vi "Clear All.vi"(8 "error in (no error)":errorcluster, 11 ".NET MSChart ref":refnum<k24>) -> ()   [LabVIEW 2014, in "XMSChart.xctl"]
uses:
  XMSChart.xctl
  System.Windows.Forms.DataVisualization
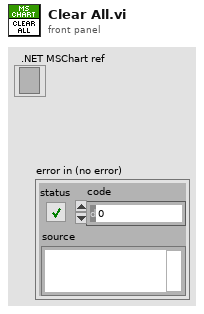
[diagram p1: front panel]
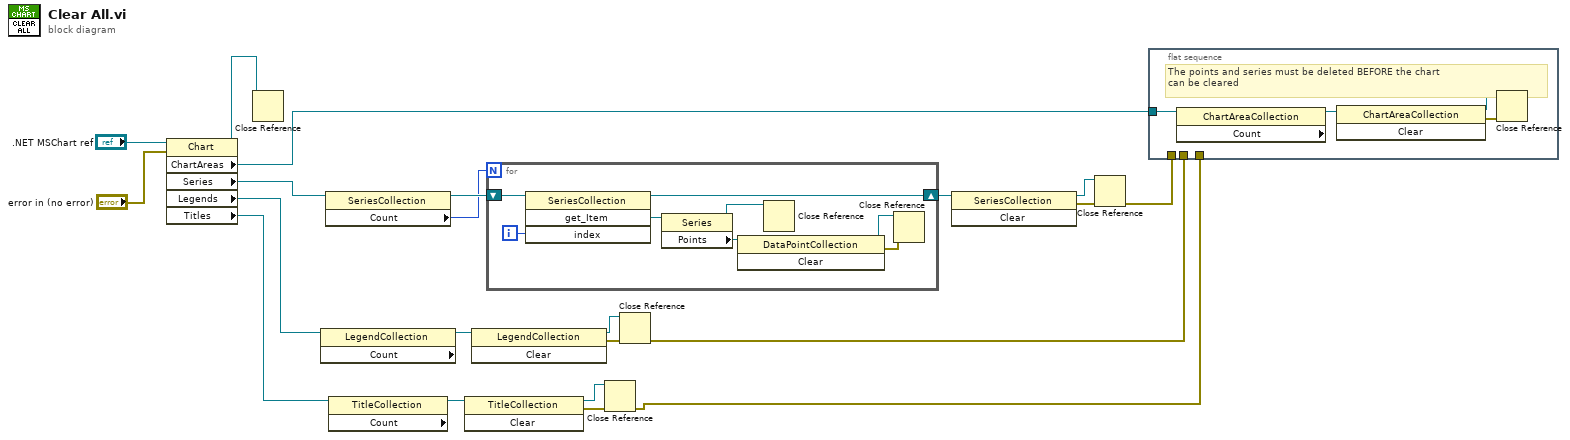
[diagram p0: block diagram]
diagram:
  n1 = property class="Chart"(reference=".NET MSChart ref", error in="error in (no error)") -> (reference out=w4:refnum<k24>, "ChartAreas"=w21:refnum<k24>, "Series"=w19:refnum<k24>, "Legends"=w10:refnum<k24>, "Titles"=w6:refnum<k24>)  [unwired: 1 out]
  n2 = Close Reference(reference=w4) -> ()  [unwired: 1 in, 1 out]
  n3 = property class="LegendCollection" props=["Count"](reference=w10) -> (reference out=w11:refnum<k24>)  [unwired: 1 in, 2 out]
  n4 = property class="SeriesCollection"(reference=w19) -> (reference out=w18:refnum<k24>, "Count"=w17:i32)  [unwired: 1 in, 1 out]
  n5 = property class="TitleCollection" props=["Count"](reference=w6) -> (reference out=w9:refnum<k24>)  [unwired: 1 in, 2 out]
  n6 = invoke class="TitleCollection" method="Clear"(reference=w9) -> (reference out=w7:refnum<k24>, error out=w8:errorcluster)  [unwired: 2 in, 1 out]
  n7 = invoke class="LegendCollection" method="Clear"(reference=w11) -> (reference out=w13:refnum<k24>, error out=w12:errorcluster)  [unwired: 2 in, 1 out]
  n8 = for {
    N: w17 -> [_]
    shift-right: [w25] -> w16
    shift-left: w18 -> [w29]
    i -> [w28]
    n9 = invoke class="SeriesCollection" method="get_Item"(reference=w29, "index"=w28) -> (reference out=w25:refnum<k24>, "get_Item"=w27:refnum<k24>)  [unwired: 2 in, 2 out]
    n10 = property class="Series"(reference=w27) -> (reference out=w24:refnum<k24>, "Points"=w26:refnum<k24>)  [unwired: 1 in, 1 out]
    n11 = invoke class="DataPointCollection" method="Clear"(reference=w26) -> (reference out=w22:refnum<k24>, error out=w23:errorcluster)  [unwired: 2 in, 1 out]
    n12 = Close Reference(reference=w24) -> ()  [unwired: 1 in, 1 out]
    n13 = Close Reference(reference=w22, error in (no error)=w23) -> ()  [unwired: 1 out]
  }
  n14 = Close Reference(reference=w7, error in (no error)=w8) -> (error out=w1:errorcluster)
  n15 = Close Reference(reference=w13, error in (no error)=w12) -> (error out=w2:errorcluster)
  n16 = invoke class="SeriesCollection" method="Clear"(reference=w16) -> (reference out=w14:refnum<k24>, error out=w15:errorcluster)  [unwired: 2 in, 1 out]
  n17 = Close Reference(reference=w14, error in (no error)=w15) -> (error out=w3:errorcluster)
  n18 = flat-sequence {
    tunnel: w21 -> [w33]
    tunnel: w3 -> [_]
    tunnel: w2 -> [_]
    tunnel: w1 -> [_]
    frame #0 {
      # "The points and series must be deleted BEFORE the chart\ncan be cleared"
      n19 = property class="ChartAreaCollection" props=["Count"](reference=w33) -> (reference out=w32:refnum<k24>)  [unwired: 1 in, 2 out]
      n20 = invoke class="ChartAreaCollection" method="Clear"(reference=w32) -> (reference out=w30:refnum<k24>, error out=w31:errorcluster)  [unwired: 2 in, 1 out]
      n21 = Close Reference(reference=w30, error in (no error)=w31) -> ()  [unwired: 1 out]
    }
  }
